vi "MCS_monocrhomator_controller_test.vi"() -> ()   [LabVIEW 2016]
uses:
  <vilib>/Instr/_visa.llb/VISA Configure Serial Port (Instr).vi
  <vilib>/Waveform/WDTFileIO.llb/Export Waveform To Spreadsheet File.vi
  <vilib>/MakerHub/Toolbox/LMH-Toolbox.lvlib
panel:
  out "RoiSum":dbl=24008.0
  in  "Main UI":T1(tab)=enum."Collect Data"
  in  "Get Position":bool
  in  "Set Zero Position":bool
  in  "Move to Target":bool
  in  "Arduino USB Port":refnum<visa-resource-name>="COM3"
  in  "Target Motor Position":i32
  out "Current Position":string="0\r\n"
  out "Settings":T2={"Range"=3520, "cftfak"=39321856, "RoiMin"=0, "RoiMax"=3520, "#Regions"=0, "Caluse"=1, "Calpoints"=0, "Param"=0, "Offset"=0, "Xdim"=0, "bitshift"=0, "Active"=1, "Roipreset"=10.0, "dummy1"=0.0, "dummy2"=0.0, "dummy3"=0.0} {"dummy3" format="%.2f"; "dummy2" format="%.2f"; "bitshift" format="%.0x"; "Active" format="%.0x"; "Offset" format="%.0x"; "Param" format="%.0x"; "dummy1" format="%.2f"; "Roipreset" format="%.2f"; "cftfak" format="%.0x"}
  in  "Maximum Scan\nPosition":dbl=3000.0
  out "Harmonics":cluster{"Y":dbl[], "Y":dbl[]}[](graph)=[{"Y"=[200.0, 300.0, 400.0, 500.0, 600.0, 700.0, 800.0, 900.0, 1000.0, 1100.0, 1200.0, 1300.0, 1400.0, 1500.0, 1600.0, 1700.0, 1800.0, 1900.0, 2000.0, 2100.0, 2200.0, 2300.0, 2400.0, 2500.0, 2600.0, 2700.0, 2800.0, 2900.0, 3000.0, 3100.0, 3200.0, 3300.0], "Y"=[0.0, 24008.0, 24008.0, 24008.0, 24008.0, 24008.0, 24008.0, 24008.0, 24008.0, 24008.0, 24008.0, 24008.0, 24008.0, 24008.0, 24008.0, 24008.0, 24008.0, 24008.0, 24008.0, 24008.0, 24008.0, 24008.0, 24008.0, 24008.0, 24008.0, 24008.0, 24008.0, 24008.0, 24008.0, 24008.0, 24008.0, 24008.0]}]
  in  "Start Scan":bool
  out "Spectrum":u32[](graph)
  in  "State":T3(ring)=enum."Move Grating"
  out "Grating Position":i16=3300
  in  "Step Size":i32=100
  in  "Sweeps":i32
  out "CHN Status":T4={"Started"=0, "Maxval"=3001, "Runtime"=0.018000000000000002, "Fifo full"=0.0, "TotalSum"=24008.0, "RoiSum"=24008.0, "Roirate"=0.0, "Sweeps"=3001.0, "Starts"=3001.0, "Dummy"=0.0} {"Dummy" format="%.2f"; "Starts" format="%.2f"; "Sweeps" format="%.2f"; "Roirate" format="%.2f"; "RoiSum" format="%.2f"; "TotalSum" format="%.2f"; "Fifo full" format="%.2f"; "Runtime" format="%.2f"}
  in  "Photoelectron Spectra Destination":path=path "C:/Users/cj09d/Desktop/SpectraTest/Today"
  out "Halt Confirmation":string="OK"
  out "MCSADat Error":i32
  in  "Spectrum #":i32
  out "Arduino Response":string="1600\r\n"
  out "Sent Message":string="M003300#"
  in  "Stop":bool
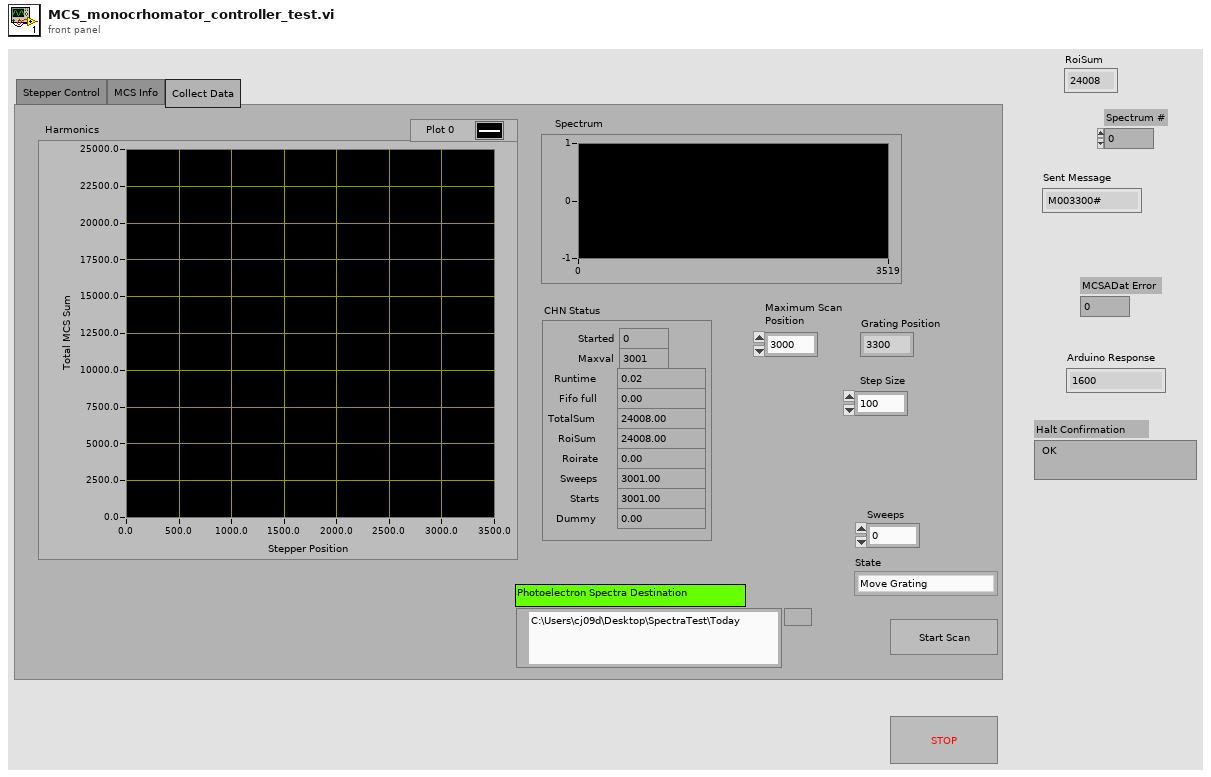
[diagram p1: front panel]
types:
  T1 = enum32{"Stepper Control", "MCS Info", "Collect Data"}
  T2 = cluster{"Range":i32, "cftfak":i32, "RoiMin":i32, "RoiMax":i32, "#Regions":i32, "Caluse":i32, "Calpoints":i32, "Param":i32, "Offset":i32, "Xdim":i32, "bitshift":i32, "Active":i32, "Roipreset":dbl, "dummy1":dbl, "dummy2":dbl, "dummy3":dbl}
  T3 = enum16{"Start", "Move Grating", "Start MCS", "Collect Data", "Stop MCS", "Save Data", "Stop"}
  T4 = cluster{"Started":i32, "Maxval":u32, "Runtime":dbl, "Fifo full":dbl, "TotalSum":dbl, "RoiSum":dbl, "Roirate":dbl, "Sweeps":dbl, "Starts":dbl, "Dummy":dbl}
  T5 = enum16{"open", "replace", "create", "open or create", "replace or create", "replace or create with confirmation"}
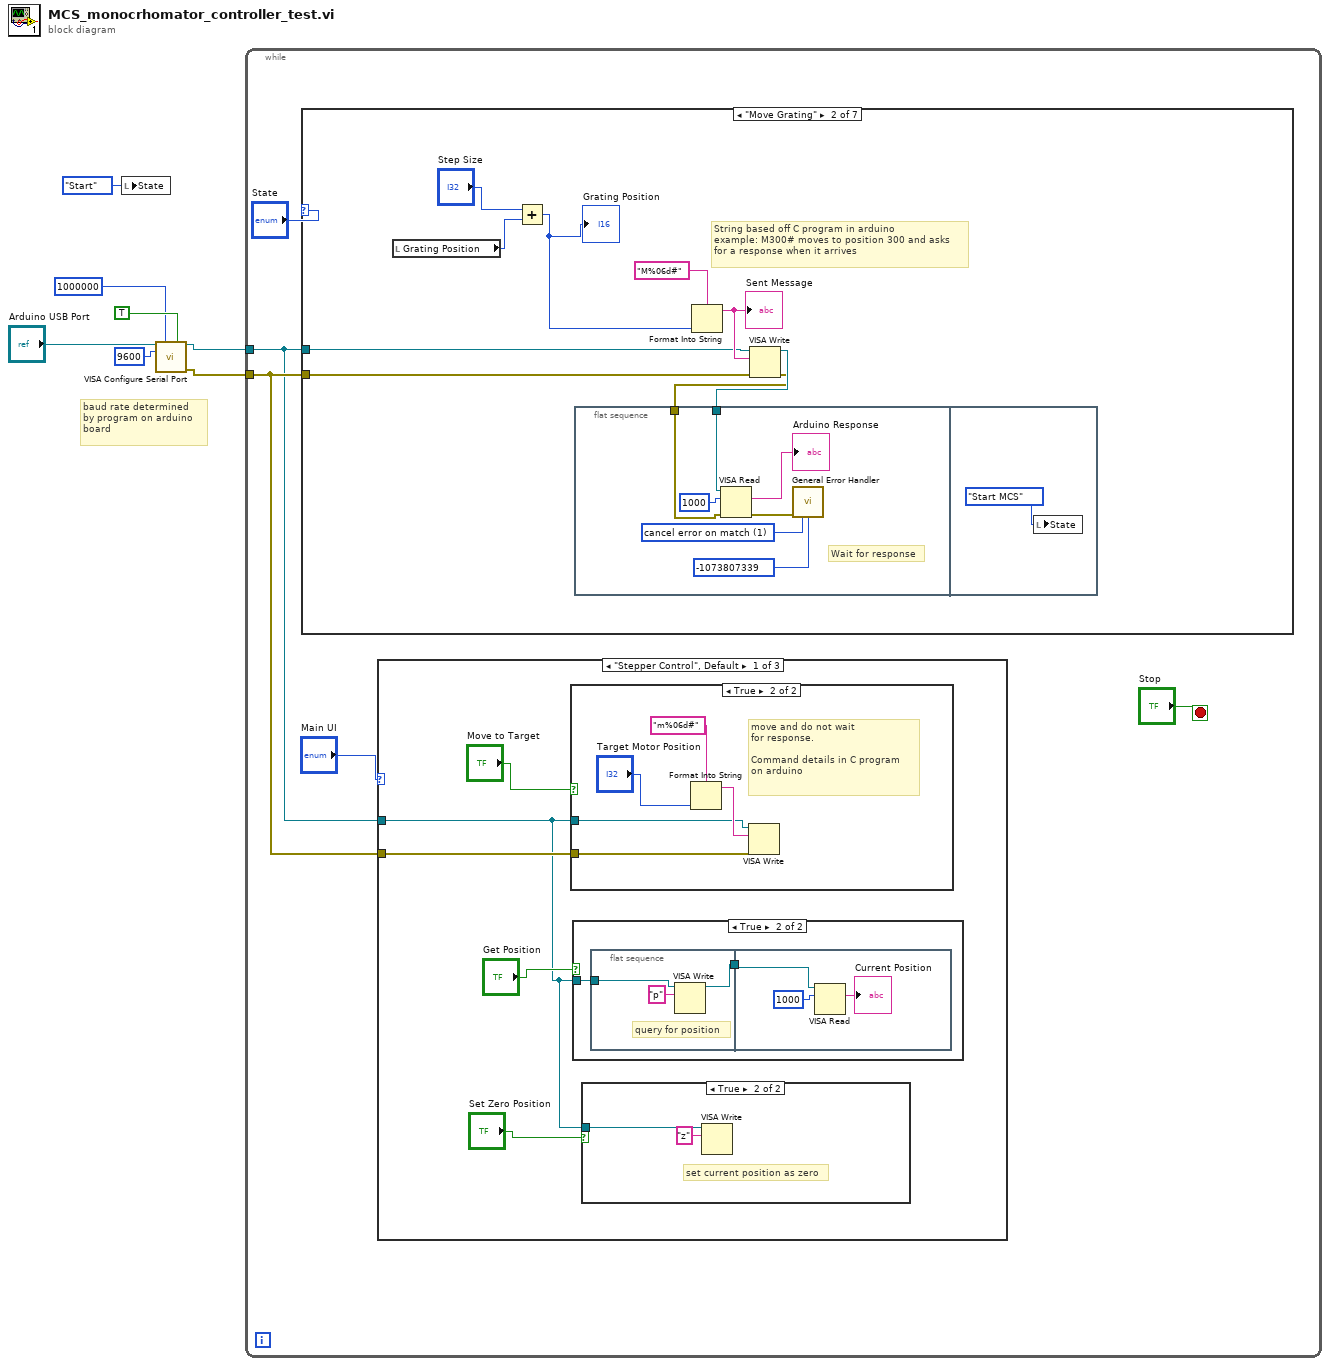
[diagram p0: block diagram]
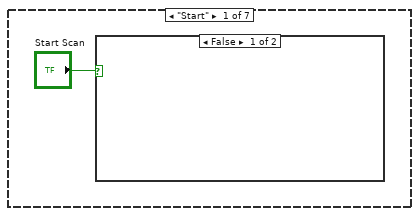
[diagram p7: hidden frame]
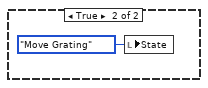
[diagram p8: hidden frame]
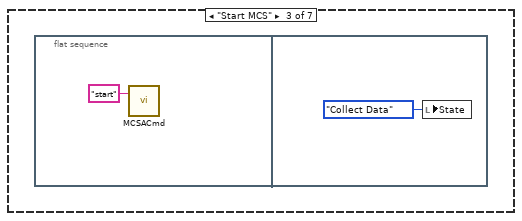
[diagram p9: hidden frame]
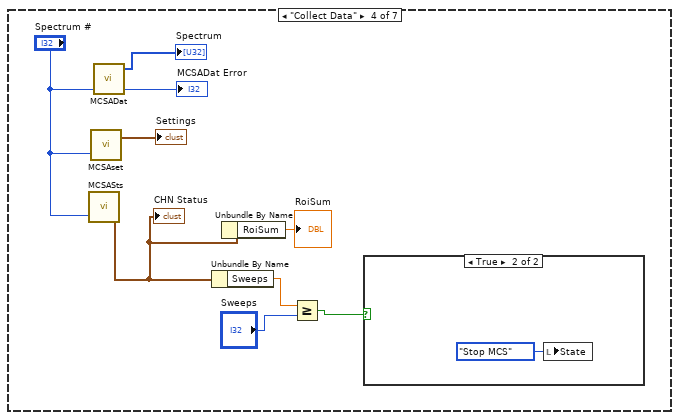
[diagram p10: hidden frame]
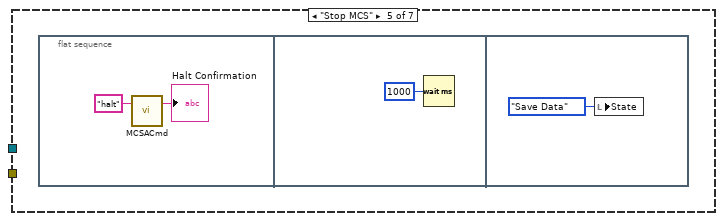
[diagram p12: hidden frame]
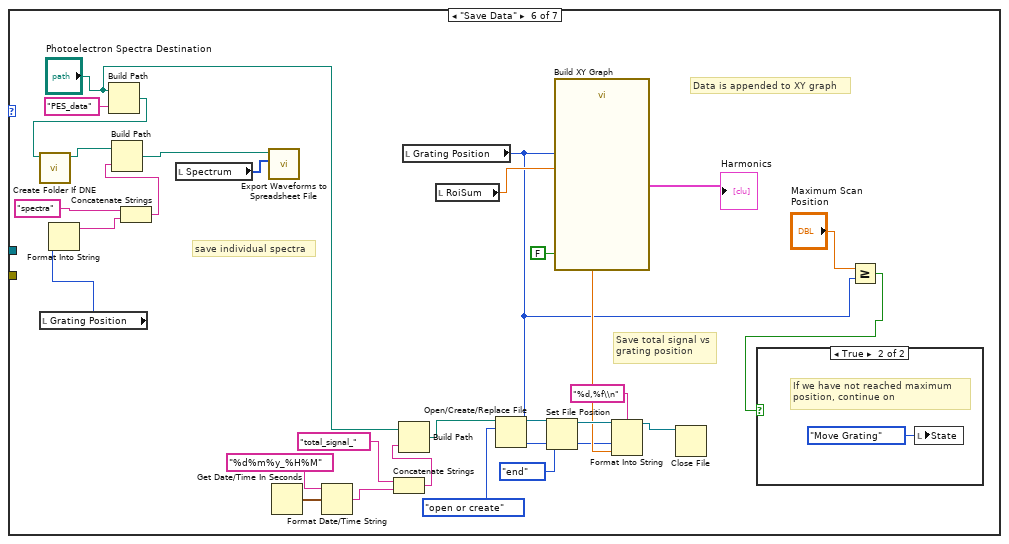
[diagram p13: hidden frame]
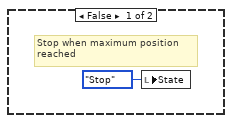
[diagram p14: hidden frame]
diagram:
  # "baud rate determined\nby program on arduino\nboard"
  n1 = local write "State"(T3."Start" ("State")) -> ()
  n2 = call-poly "VISA Configure Serial Port"("VISA resource name"="Arduino USB Port", "timeout (10sec)"=u32 1000000, "Enable Termination\nChar (T)"=TRUE, "baud rate (9600)"=u32 9600 ("baud rate")) -> ("VISA resource name out"=w1:refnum<visa-resource-name>, "error out"=w2:errorcluster)  [unwired: 6 in, 4 out]
  n3 = while {
    tunnel: w1 -> [w8]
    tunnel: w2 -> [w9]
    stop <- "Stop" stop-if-true
    n4 = case shown="\"Move Grating\"" "State" {
      tunnel: w8 -> [_ w41 _ _ _ _ _]
      tunnel: w9 -> [_ w40 _ _ _ _ _]
      frame "Start" {
        n5 = case shown="False" "Start Scan" {
          frame False {
          }
          frame True {
            n6 = local write "State"(T3."Move Grating" ("State")) -> ()
          }
        }
      }
      frame "Move Grating" {
        # "String based off C program in arduino\nexample: M300# moves to position 300 and asks\nfor a response when it arrives"
        n7 = local read "Grating Position"() -> (w38:i16)
        n8 = Add(x="Step Size", y=w38) -> (x+y=w35:i32)
        "Grating Position" <- w35
        n9 = flat-sequence {
          tunnel: w37 -> [w45]
          tunnel: w36 -> [w44]
          frame #0 {
            w48 = 1 items=["no exception", "cancel error on match", "set error on match"] ("[exception action] (none:0)")
            # "Wait for response"
            n10 = VISA Read(VISA resource name=w45, byte count=1000, error in (no error)=w44) -> (read buffer=→"Arduino Response":string, error out=w50:errorcluster)  [unwired: 2 out]
            n11 = call <vilib>:"General Error Handler.vi"("error in (no error)"=w50, "[exception action] (none:0)"=w48, "[exception code]"=-1073807339) -> ()  [unwired: 8 in, 5 out]
          }
          frame #1 {
            n12 = local write "State"(T3."Start MCS" ("State")) -> ()
          }
        }
        n13 = Format Into String(format string="M%06d#", w35) -> (resulting string=w42:string)  [unwired: 2 in, 1 out]
        "Sent Message" <- w42
        n14 = VISA Write(VISA resource name=w41, write buffer=w42, error in (no error)=w40) -> (VISA resource name out=w37:refnum<visa-resource-name>, error out=w36:errorcluster)  [unwired: 1 out]
      }
      frame "Start MCS" {
        n15 = flat-sequence {
          frame #0 {
            n16 = call "MCSACmd.vi"("Command"="start") -> ()  [unwired: 2 in, 1 out]
          }
          frame #1 {
            n17 = local write "State"(T3."Collect Data" ("State")) -> ()
          }
        }
      }
      frame "Collect Data" {
        n18 = call "MCSASts.vi"("CHN #"="Spectrum #") -> ("CHN Status"=w55:T4)  [unwired: 1 in, 1 out]
        "CHN Status" <- w55
        n19 = call "MCSAset.vi"("Spect #"="Spectrum #") -> ("Settings"=→"Settings":T2)  [unwired: 1 in, 1 out]
        n20 = call "MCSADat.vi"("Spectrum #"="Spectrum #") -> ("MCSADat Error"=→"MCSADat Error":i32, "Data"=→"Spectrum":u32[])  [unwired: 2 in, 1 out]
        n21 = Unbundle By Name(w55) -> ("Sweeps"=w58:dbl)
        n22 = Unbundle By Name(w55) -> ("RoiSum"=→"RoiSum":dbl)
        n23 = Greater Or Equal?(x=w58, y="Sweeps") -> (x >= y?=w56:bool)
        n24 = case shown="True" w56 {
          frame False {
            # "Do nothing, continue\ncollecting data"
          }
          frame True {
            n25 = local write "State"(T3."Stop MCS" ("State")) -> ()
          }
        }
      }
      frame "Stop MCS" {
        n26 = flat-sequence {
          frame #0 {
            n27 = call "MCSACmd.vi"("Command"="halt") -> ("Response"=→"Halt Confirmation":string)  [unwired: 2 in]
          }
          frame #1 {
            n28 = Wait (ms)(milliseconds to wait=u32 1000) -> ()  [unwired: 1 out]
          }
          frame #2 {
            n29 = local write "State"(T3."Save Data" ("State")) -> ()
          }
        }
      }
      frame "Save Data" {
        # "Data is appended to XY graph"
        # "Save total signal vs\ngrating position"
        # "save individual spectra"
        n30 = local read "Grating Position"() -> (w92:i16)
        n31 = Format Into String(w92) -> (resulting string=w93:string)  [unwired: 3 in, 1 out]
        n32 = Build Path(base path="Photoelectron Spectra Destination", name or relative path="PES_data") -> (appended path=w89:path)
        n33 = call <vilib>:"Create Folder If DNE.vi"("Folder Path"=w89) -> ("Dup Path"=w88:path)  [unwired: 9 in, 1 out]
        n34 = Concatenate Strings("spectra" ("string"), w93) -> (w95:string)
        n35 = Build Path(base path=w88, name or relative path=w95) -> (appended path=w87:path)
        n36 = local read "Spectrum"() -> (w91:u32[])
        n37 = call-poly <vilib>:"Export Waveforms to Spreadsheet File.vi"("waveform"=w91, "file path (dialog if empty)"=w87) -> ()  [unwired: 8 in, 2 out]
        n38 = Get Date/Time In Seconds() -> (seconds since 1Jan1904=w83:timestamp)
        n39 = Format Date/Time String(time format string (%c)="%d%m%y_%H%M", seconds (now)=w83) -> (date/time string=w82:string)  [unwired: 1 in]
        n40 = Concatenate Strings("total_signal_" ("string"), w82) -> (w79:string)
        n41 = Build Path(base path="Photoelectron Spectra Destination", name or relative path=w79) -> (appended path=w78:path)
        n42 = local read "Grating Position"() -> (w69:i16)
        n43 = local read "RoiSum"() -> (w74:dbl)
        n44 = Open/Create/Replace File(file path (use dialog)=w78, operation (0:open)=T5."open or create") -> (refnum out=w77:refnum<file>)  [unwired: 4 in, 2 out]
        n45 = Set File Position(refnum=w77, from (0:start)=enum16{"start", "end", "current"}."end") -> (refnum out=w75:refnum<file>)  [unwired: 2 in, 1 out]
        n46 = call "Build XY Graph"("Reset"=FALSE, "Y Input"=w74, "X Input"=w69) -> ("XY Graph"=→"Harmonics":cluster{"X":dbl[], "Y":dbl[]}[])  [unwired: 7 in, 1 out]
        n47 = Format Into String(format string="%d,%f\\n", initial string=w75, w69, w74) -> (resulting string=w72:refnum<file>)  [unwired: 1 in, 1 out]
        n48 = Close File(refnum=w72) -> ()  [unwired: 1 in, 2 out]
        n49 = Greater Or Equal?(x="Maximum Scan\nPosition", y=w69) -> (x >= y?=w68:bool)
        n50 = case shown="True" w68 {
          frame False {
            # "Stop when maximum position\nreached"
            n51 = local write "State"(T3."Stop" ("State")) -> ()
          }
          frame True {
            # "If we have not reached maximum\nposition, continue on"
            n52 = local write "State"(T3."Move Grating" ("State")) -> ()
          }
        }
      }
      frame "Stop", Default {
      }
    }
    n53 = case shown="\"Stepper Control\", Default" "Main UI" {
      tunnel: w9 -> [w15 _ _]
      tunnel: w8 -> [w13 _ _]
      frame "Stepper Control", Default {
        n54 = case shown="True" "Move to Target" {
          tunnel: w15 -> [_ w29]
          tunnel: w13 -> [_ w28]
          frame False {
          }
          frame True {
            # "move and do not wait\nfor response.\n\nCommand details in C program\non arduino"
            n55 = Format Into String(format string="m%06d#", "Target Motor Position") -> (resulting string=w31:string)  [unwired: 2 in, 1 out]
            n56 = VISA Write(VISA resource name=w28, write buffer=w31, error in (no error)=w29) -> ()  [unwired: 3 out]
          }
        }
        n57 = case shown="True" "Get Position" {
          tunnel: w13 -> [_ w20]
          frame False {
          }
          frame True {
            n58 = flat-sequence {
              tunnel: [w24] -> w21
              tunnel: w20 -> [w22]
              tunnel: w21 -> [w26]
              frame #0 {
                # "query for position"
                n59 = VISA Write(VISA resource name=w22, write buffer="p") -> (VISA resource name out=w24:refnum<visa-resource-name>)  [unwired: 1 in, 2 out]
              }
              frame #1 {
                n60 = VISA Read(VISA resource name=w26, byte count=1000) -> (read buffer=→"Current Position":string)  [unwired: 1 in, 3 out]
              }
            }
          }
        }
        n61 = case shown="True" "Set Zero Position" {
          tunnel: w13 -> [_ w18]
          frame False {
          }
          frame True {
            # "set current position as zero"
            n62 = VISA Write(VISA resource name=w18, write buffer="z") -> ()  [unwired: 1 in, 3 out]
          }
        }
      }
      frame "MCS Info" {
        # "Ensure MCS6A.exe is running and that the 32/64 bit version of LabView matches the version of the MCS\nsoftware running, most setup done through that program\n\nIn particular set a Sweeps Preset under Hardware Options to be the desired sweeps + 1"
      }
      frame "Collect Data" {
        # "This state is continuously running based on the State variable\nSee large above case structure"
      }
    }
  }
